vi "Init_Test.vi"(8 "error in (no error)":errorcluster caption="entrée d'erreur (pas d'erreur)", 11 "Flash_Jlink en entrée":refnum<class "P2265_SwitchOn_Test.lvclass">) -> (0 "error out":errorcluster caption="sortie d'erreur", 3 "Flash_Jlink en sortie":refnum<class "P2265_SwitchOn_Test.lvclass">)   [LabVIEW 2020, in "Library Test.lvlib" / "P2265_SwitchOn_Test.lvclass"]
uses:
  P2265_SwitchOn_Test.lvclass
  C:/Users/ngarcin/OneDrive - Altyor/Standard TB/Class/Test/Test (Default)/Test (Default).lvclass
  Commun VI/TypeDef/Commande Test/Commande Type Test.ctl
  Commun VI/TypeDef/Commande Test/Commande Value Type.ctl
  Commun VI/TypeDef/Commande Relay_Board/Parameter Relay_Board.ctl
  Relay_Board/Relay_Board (Default)/Class Relay_Board (Default).lvclass
  JSON API/JSON Value/Set from JSON string.vi
  JSON API/Variant JSON/Variant to JSON.vi
  JSON API/JSON Value/Get Item by name array.vi
  Test_Wtih_Instr/Test_With_Inst.lvclass
  Instrument/Instrument (Default)/Class Instrument (Default).lvclass
  JSON API/JSON Value/JSON Value.lvclass
  P2265_SwitchOn_Test.lvclass/P2265_SwitchOn_Test.ctl
  Commun VI/Library Commun.lvlib
  JSON API/Get Polymorphic/JSON GetSet.lvlib
  JSON API/Variant JSON/Variant JSON.lvlib
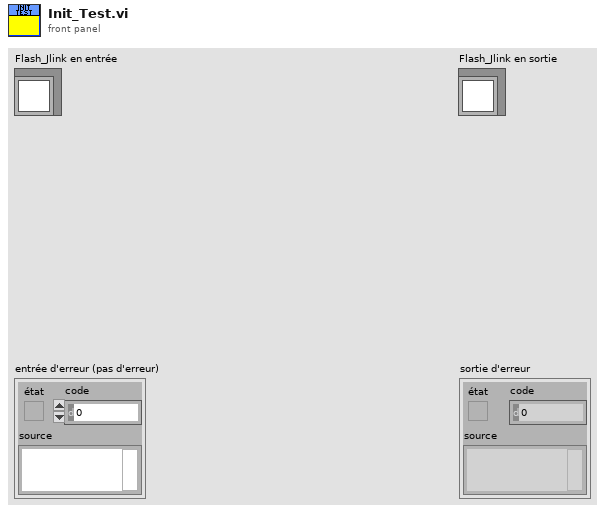
[diagram p1: front panel]
types:
  T1 = typedef "Library Commun.lvlib/Parameter Relay_Board.ctl" = cluster{"Device_Com_Port":string, "Address Board":string, "Tab_Num_Relay":u8[], "Parameter Class Relay_Board":refnum<class "Class Relay_Board (Default).lvclass">}
  T2 = typedef "Library Commun.lvlib/Commande Value Type.ctl" = enum16{"None", "String", "Number", "Timestamp", "Boolean", "Array"}
  T3 = typedef "Library Commun.lvlib/Commande Type Test.ctl" = enum16{"Function", "Test", "Calculation"}
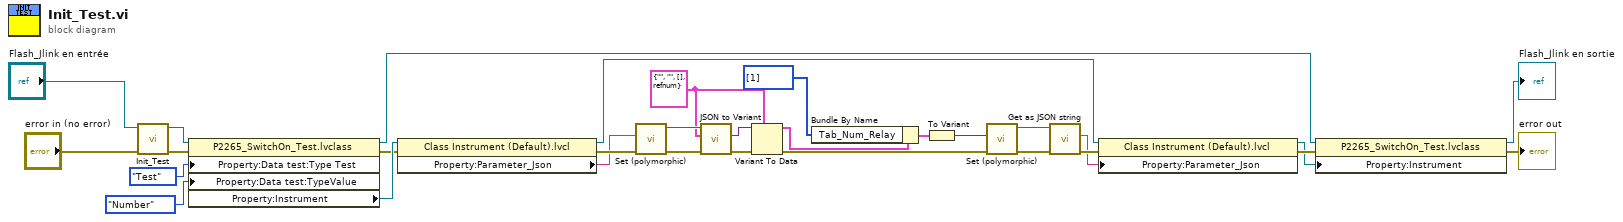
[diagram p0: block diagram]
diagram:
  w19 = T1 {"Device_Com_Port"="", "Address Board"="", "Tab_Num_Relay"=[], "Parameter Class Relay_Board"=refnum} ("Parameter")
  n1 = call-parent "Init_Test.vi"("error in (no error)"="error in (no error)", "Test_With_Inst en entrée"="Flash_Jlink en entrée") -> ("error out"=w26:errorcluster, "Test_With_Inst en sortie"=w27:refnum<class "P2265_SwitchOn_Test.lvclass">)  [unwired: 8 in]
  n2 = property class="P2265_SwitchOn_Test.lvclass"(reference=w27, error in=w26, "Property:Data test:Type Test"=Commande_Type_Test."Test" ("Type Test"), "Property:Data test:TypeValue"=Commande_Value_Type."Number" ("TypeValue")) -> (reference out=w2:refnum<class "P2265_SwitchOn_Test.lvclass">, error out=w6:errorcluster, "Property:Instrument"=w8:refnum<class "Class Instrument (Default).lvclass">)
  n3 = property class="Class Instrument (Default).lvcl"(reference=w8, error in=w6) -> (reference out=w7:refnum<class "Class Instrument (Default).lvclass">, error out=w20:errorcluster, "Property:Parameter_Json"=w10:string)
  n4 = call-poly "Set (polymorphic).vi"("error in (no error)"=w20, "JSON stream"=w10) -> ("error out"=w23:errorcluster, "JSON Value out"=w21:refnum<class "JSON Value.lvclass">)  [unwired: 7 in, 1 out]
  n5 = call "JSON to Variant.vi"("error in (no error)"=w23, "Variant (Data Type)"=w19, "JSON Value"=w21) -> ("error out"=w22:errorcluster, "Variant out"=w24:variant)  [unwired: 7 in]
  n6 = Variant To Data(error in=w22, type=w19, Variant=w24) -> (data=w18:T1, error out=w13:errorcluster)
  n7 = Bundle By Name(cluster=w18, "Tab_Num_Relay"=u8[] [1]) -> (w11:T1)
  n8 = To Variant(anything=w11) -> (Variant=w16:variant)
  n9 = call-poly "Set (polymorphic).vi"("error in (no error)"=w13, "Variant"=w16) -> ("error out"=w14:errorcluster, "JSON Value out"=w15:refnum<class "JSON Value.lvclass">)  [unwired: 8 in]
  n10 = call "Get as JSON string.vi"("error in (no error)"=w14, "JSON Value in"=w15) -> ("error out"=w12:errorcluster, "<JSON>"=w9:string)  [unwired: 8 in]
  n11 = property class="Class Instrument (Default).lvcl"(reference=w7, error in=w12, "Property:Parameter_Json"=w9) -> (reference out=w3:refnum<class "Class Instrument (Default).lvclass">, error out=w5:errorcluster)
  n12 = property class="P2265_SwitchOn_Test.lvclass"(reference=w2, error in=w5, "Property:Instrument"=w3) -> (reference out=→"Flash_Jlink en sortie":refnum<class "P2265_SwitchOn_Test.lvclass">, error out=→"error out":errorcluster)
